vi "Scan_Hopping_percentDecrease_VUW.vi"() -> ()   [LabVIEW 2023]
uses:
  Sub_Vi/TypeDefs/Settings.ctl
  Sub_Vi/TypeDefs/ChangeOnFly.ctl
  Sub_Vi/TypeDefs/Display.ctl
  Settings.vi
panel:
  out "Precent Change for feedback (percent) 2":dbl=2.0
  in  "StopCond_GreaterThan? 2":bool
  in  "Display Cluster":T1
  in  "ChangeonFly":T2
  in  "SettingsCluster":T3={"Sample Rate (us)"=1, "Samples Per Data Point (int, power of 2)"=1000, "DistanceToBulk (um)"=-1.0, "HoldTimeScaler"=40000, "SaveData"=TRUE, "DistanceToBulk (um) 2"=-1.0, "DistanceToBulk (um) 3"=-1.0}
  in  "Feedback Type":T4(ring)=enum."Current 1"
  in  "StopCond_GreaterThan?":bool=TRUE
  in  "Approach Rate (um/s)":dbl=0.15
  in  "Retract Rate (um/s)":dbl=1.0
  in  "Hopping Distance (um)":dbl=1.0
  in  "Z End height (um)":dbl
  in  "Distance To Retract (um)":dbl=5.0
  in  "Upper dZ limit":i32=8
  in  "Precent Change for feedback (percent)":dbl=2.0
  in  "P":fxp<+/-,32,1>=0.029999999795109034 format="%.32g"
  in  "X Center (um)":dbl=100.0 min=0.0 max=300.0
  in  "Y Center (um)":dbl=100.0 min=0.0 max=300.0
  in  "Y Width (um)":dbl=10.0
  in  "X Width (um)":dbl=10.0
  in  "Scan Rate (um/s)":dbl=5.0
  in  "Voltage to Electrode (V)":dbl=-0.4
  in  "Z Start height (um)":dbl=150.0
  in  "Start scan Button":bool
  in  "Stop":bool
  in  "Pause":bool
  in  "Start Scanning Button":bool
  out "Y end":dbl
  out "X end":dbl
  out "X start":dbl
  out "Y start":dbl
  in  "Tab Control 4":enum32{"AC Approach 2"}(tab)
  out "t vs C1":dbl[](graph)
  out "Z vs C1":cluster{"Y":dbl[], "Y":dbl[]}[](graph)
  # "Approach  Settings"
  # "Feedback  Settings"
  # "Scan  Settings"
  # "Define Scan area \nAbout centre"
  # "Settings"
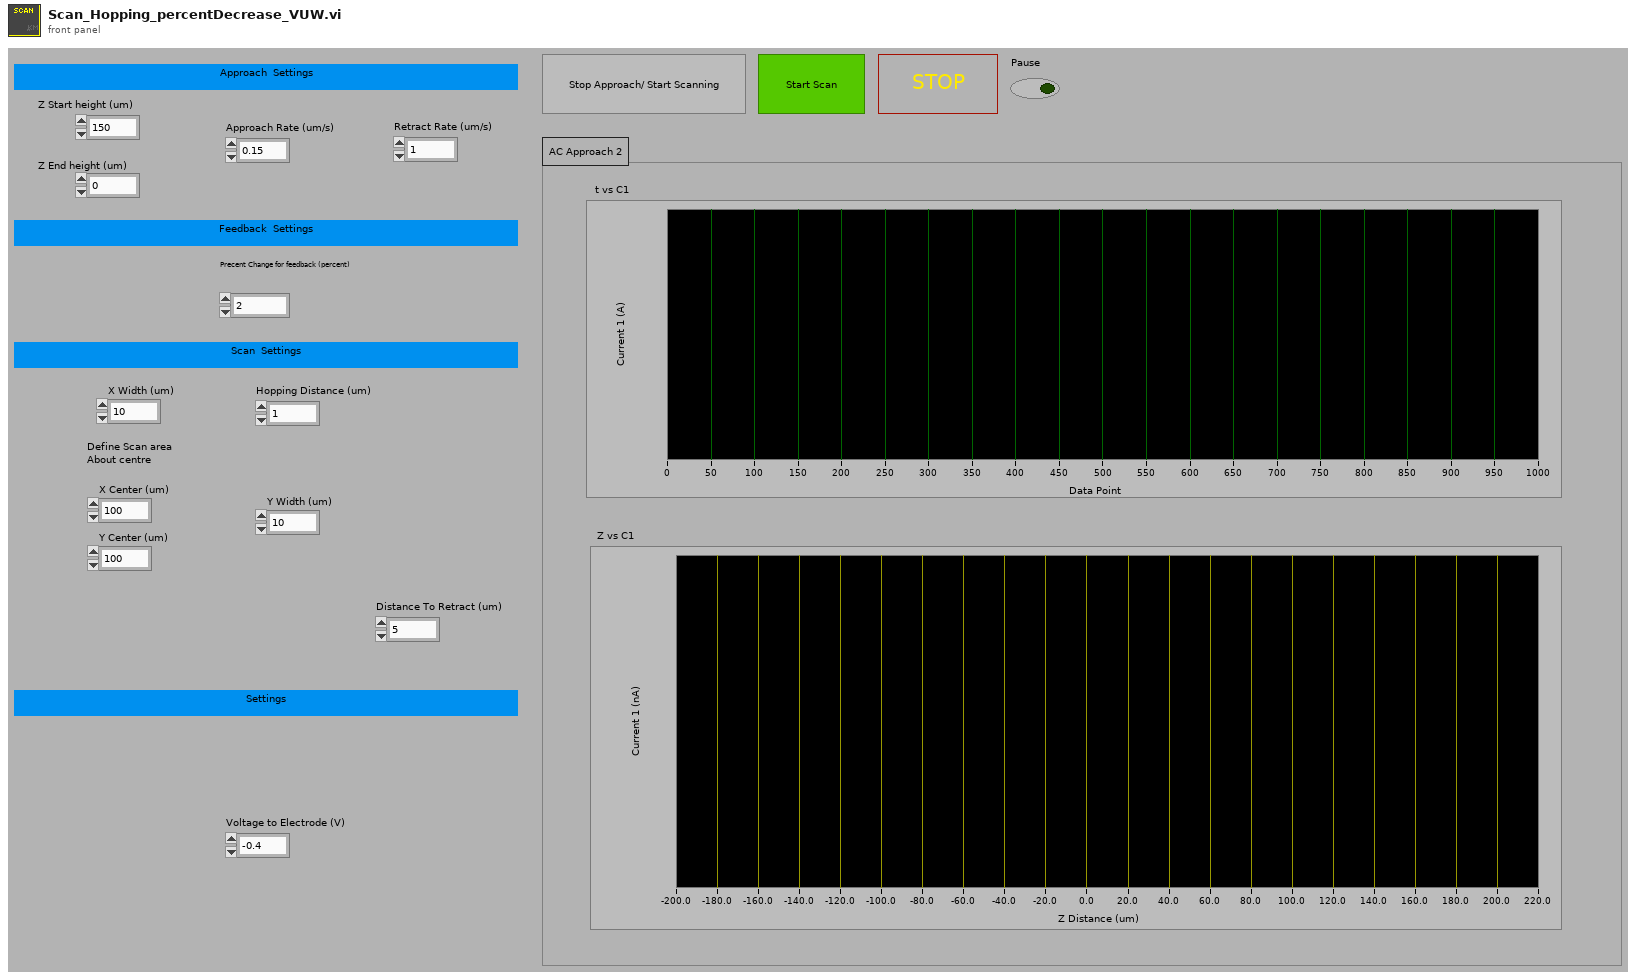
[diagram p1: front panel]
types:
  T1 = typedef "Display.ctl" = cluster{"X":refnum<vi>, "Y":refnum<vi>, "Z":refnum<vi>, "Amp":refnum<vi>, "Phase":refnum<vi>, "t vs Z":refnum<vi>, "t vs C1":refnum<vi>, "t vs C2":refnum<vi>, "t vs C3":refnum<vi>, "t vs Amp":refnum<vi>, "t vs Phase":refnum<vi>, "t vs X":refnum<vi>, "t vs Y":refnum<vi>, "Z vs C1":refnum<vi>, "Z vs C2":refnum<vi>, "Z vs C3":refnum<vi>, "V vs C1":refnum<vi>, "V vs C2":refnum<vi>, "V vs C3":refnum<vi>, "X/Y/Z F":refnum<vi>, "X/Y/Z R":refnum<vi>, "X/Y/C1 F":refnum<vi>, "X/Y/C1 R":refnum<vi>, "X/Y/C2 F":refnum<vi>, "X/Y/C2 R":refnum<vi>, "X/Y/C3 F":refnum<vi>, "X/Y/C3 R":refnum<vi>, "NumberOfLines":u16, "um Per Pixel":dbl, "um Per Line":dbl, "X Center":dbl, "Hop X/Y/Z":refnum<vi>, "Hop X/Y/C1":refnum<vi>, "Hop X/Y/C2":refnum<vi>, "Hop X/Y/C3":refnum<vi>, "X Width":dbl, "Y Width":dbl, "Hopping Distance":dbl, "V2 vs C1":refnum<vi>, "V vs Phase":refnum<vi>, "Y Center":dbl, "Number of Pixels":dbl, "V2 vs C2":refnum<vi>, "V2 vs C3":refnum<vi>, "V vs y":refnum<vi>, "V2 vs y":refnum<vi>, "Z vs Amp":refnum<vi>, "Z vs Phase":refnum<vi>}
  T2 = typedef "ChangeOnFly.ctl" = cluster{"Stop (boolean)":refnum<vi>, "Pause (boolean)":refnum<vi>, "EndCurrentLine (boolean)":refnum<vi>, "max movement per update step (Interger, nm)":refnum<vi>, "P (float, arb)":refnum<vi>, "Feedback set point (double, Amps)":refnum<vi>, "Voltage (double, V)":refnum<vi>, "Feedback set point 2 (double, Amps)":refnum<vi>, "Stop on Greater Than 2? (boolean)":refnum<vi>, "Stop on Greater Than? (boolean)":refnum<vi>, "Voltage 2 (double, V)":refnum<vi>, "Feedback Type (enum)":refnum<vi>, "Feedback Type 2 (enum)":refnum<vi>}
  T3 = typedef "Settings.ctl" = cluster{"Sample Rate (us)":u32, "Samples Per Data Point (int, power of 2)":i16, "DistanceToBulk (um)":dbl, "HoldTimeScaler":u64, "SaveData":bool, "DistanceToBulk (um) 2":dbl, "DistanceToBulk (um) 3":dbl}
  T4 = enum16{"AC Magnitude", "Current 1", "Current 2", "Phase"}
  T5 = cluster{"Scan Rate (um/s)":dbl, "X Start":dbl, "X End":dbl, "Y Start":dbl, "Y End":dbl, " Z Start":dbl, "HoppingDistance":dbl, "V":dbl, "Z End":dbl, "Approach Rate Hopping (um/s)":dbl, "Retrack Rate (um/s)":dbl, "V 2":dbl, "Approach Rate (um/s)":dbl, "Hold Time START / s":dbl, "Hold Time Delta / s":dbl, "Voltage to Electrode During Retract":dbl, "Pause on First Approach?":bool}
  T6 = typedef "Current Amplifier Settings.ctl" = dbl
  T7 = typedef "WayPointCluster.ctl" = cluster{"X (um)":dbl[], "Y (um)":dbl[], "Z (um)":dbl[], "V (V)":dbl[], "X Velocity (um s-1)":dbl[], "Y Velocity (um s-1)":dbl[], "Z Velocity (um s-1)":dbl[], "V Velocity (V s-1)":dbl[], "FeedBack Type (enum)":u16[], "Move X (boolean)":bool[], "Move Y (boolean)":bool[], "Move Z (boolean)":bool[], "Move V (boolean)":bool[], "Jump V (boolean)":bool[], "Hold (boolean)":bool[], "Hold Time":u32[], "V2 (V)":dbl[], "Move V2":bool[], "V2 Velocity (V s-1)":dbl[], "Jump V2 (boolean)":bool[], "Update z Position delta (ms)":i16[], "Hold Feedback1":bool[], "Move Z PicoMotor":bool[], " Z PicoMotor Direction":bool[], "DIO0":bool[]}
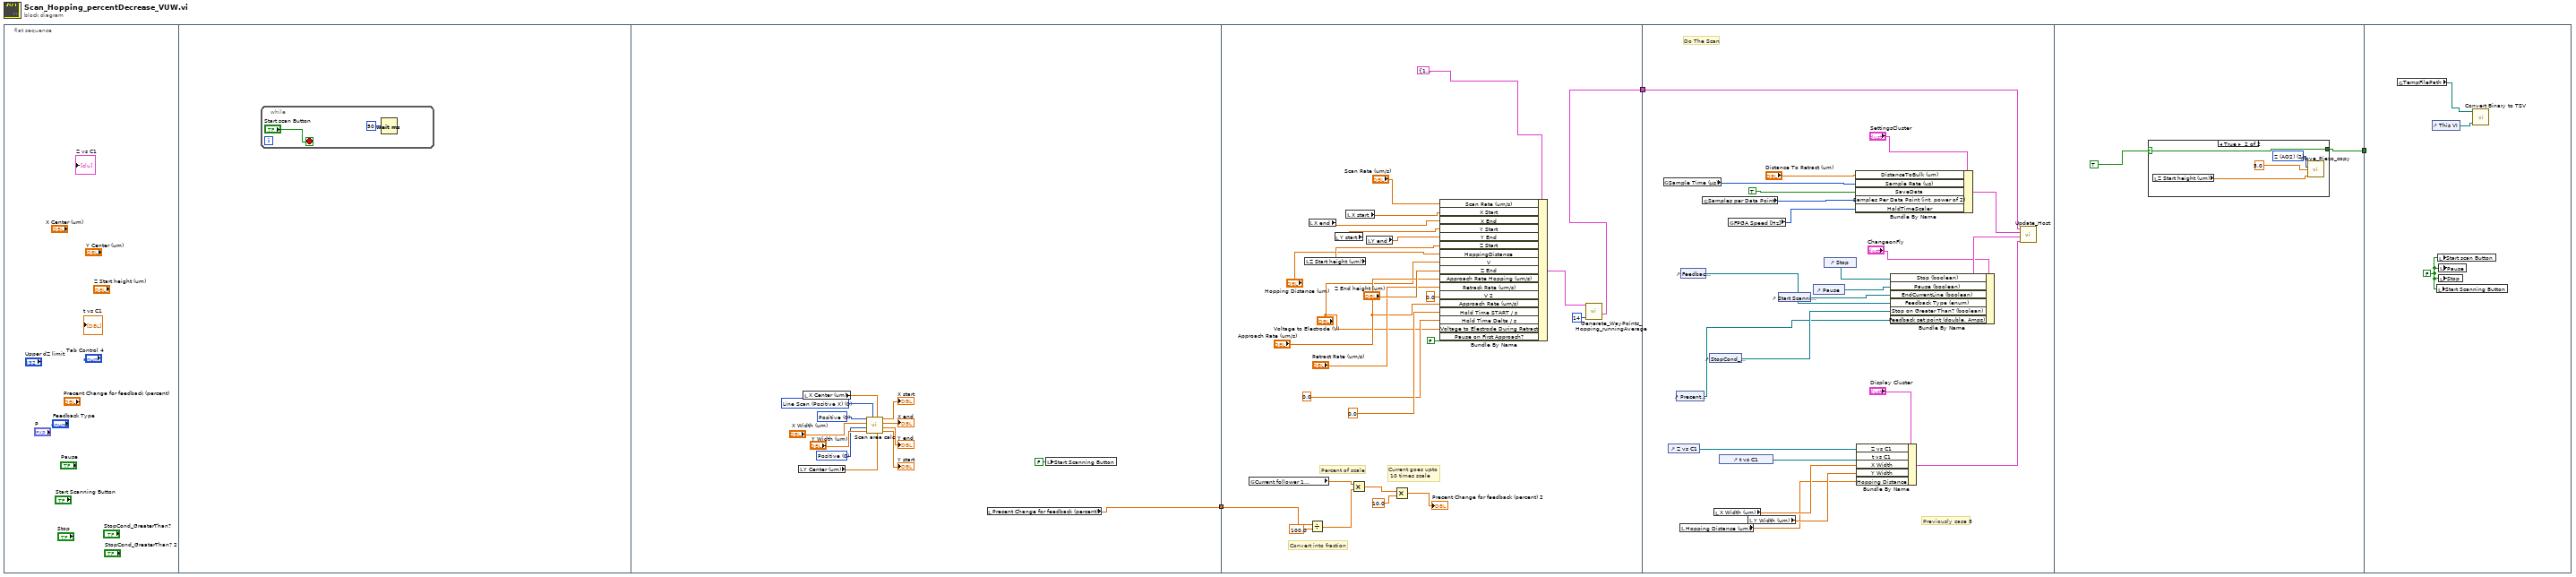
[diagram p0: block diagram]
diagram:
  n1 = flat-sequence {
    tunnel: [w6] -> w1
    tunnel: [w27] -> w3
    tunnel: w1 -> [w25]
    tunnel: w3 -> [w67]
    tunnel: [w68] -> w2
    tunnel: w2 -> [_]
    frame #0 {
    }
    frame #1 {
      n2 = while {
        stop <- "Start scan Button" stop-if-true
        n3 = Wait (ms)(milliseconds to wait=u32 50) -> ()  [unwired: 1 out]
      }
    }
    frame #2 {
      w10 = u16 0 items=["Positive", "Negative"] ("Major Axis Direction")
      w9 = u16 0 items=["Positive", "Negative"] ("Minor Axis Direction")
      w8 = u16 0 items=["Line Scan (Positive X)", "Line Scan (Negative X)", "Line Scan (Positive Y)", "Line Scan (Negative Y)"] ("Scan Type")
      n4 = local read "Y Center (um)"() -> (w18:dbl)
      n5 = local read "X Center (um)"() -> (w17:dbl)
      n6 = call "Scan area calc.vi"("Y Width"="Y Width (um)", "Major Axis Direction"=w10, "X Width"="X Width (um)", "Minor Axis Direction"=w9, "Scan Type"=w8, "Y Center"=w18, "X Center"=w17) -> ("Y start"=→"Y start":dbl, "Y end"=→"Y end":dbl, "X end"=→"X end":dbl, "X start"=→"X start":dbl)
      n7 = local read "Precent Change for feedback (percent)"() -> (w6:dbl)
      n8 = local write "Start Scanning Button"(FALSE ("Start Scanning Button")) -> ()
    }
    frame #3 {
      # "Current goes upto\n 10 times scale"
      # "Percent of scale"
      # "Convert into fraction"
      n9 = global read "Settings.vi" "Current follower 1\n (AI-3)"() -> (w22:T6)
      n10 = local read "Z Start height (um)"() -> (w38:dbl)
      n11 = local read "X end"() -> (w41:dbl)
      n12 = Divide(x=w25, y=100.0) -> (x/y=w23:dbl)
      n13 = local read "Y start"() -> (w40:dbl)
      n14 = local read "X start"() -> (w42:dbl)
      n15 = Multiply(x=w22, y=w23) -> (x*y=w21:T6)
      n16 = local read "Y end"() -> (w39:dbl)
      n17 = Multiply(x=w21, y=10.0) -> (x*y=→"Precent Change for feedback (percent) 2":T6)
      n18 = Bundle By Name(cluster=T5 {"Scan Rate (um/s)"=15.0, "X Start"=15.0, "X End"=15.0, "Y Start"=15.0, "Y End"=15.0, " Z Start"=15.0, "HoppingDistance"=1.0, "V"=15.0, "Z End"=15.0, "Approach Rate Hopping (um/s)"=15.0, "Retrack Rate (um/s)"=15.0, "V 2"=15.0, "Approach Rate (um/s)"=15.0, "Hold Time START / s"=15.0, "Hold Time Delta / s"=15.0, "Voltage to Electrode During Retract"=0.0, "Pause on First Approach?"=FALSE} ("Input Cluster"), "Scan Rate (um/s)"="Scan Rate (um/s)", "X Start"=w42, "X End"=w41, "Y Start"=w40, "Y End"=w39, "Z Start"=w38, "HoppingDistance"="Hopping Distance (um)", "V"="Voltage to Electrode (V)", "Z End"="Z End height (um)", "Approach Rate Hopping (um/s)"="Approach Rate (um/s)", "Retrack Rate (um/s)"="Retract Rate (um/s)", "V 2"=0.0, "Approach Rate (um/s)"="Approach Rate (um/s)", "Hold Time START / s"=0.0 ("IT Time /s"), "Hold Time Delta / s"=0.0 ("IT Time Delta /s"), "Voltage to Electrode During Retract"="Voltage to Electrode (V)", "Pause on First Approach?"=FALSE) -> (w28:T5)
      n19 = call "Generate_WayPoints_Hopping_runningAverage.vi"("element"=u16 14, "Input Cluster"=w28) -> ("output cluster"=w27:T7)  [unwired: 9 in]
    }
    frame #4 {
      # "Previously case 8"
      # "Do The Scan"
      n20 = global read "Settings.vi" "Sample Time (µs)"() -> (w50:u32)
      n21 = control-ref of="Z vs C1"() -> (w59:refnum<vi>)
      n22 = control-ref of="Precent Change for feedback (percent) 2"() -> (w45:refnum<vi>)
      n23 = local read "Hopping Distance (um)"() -> (w56:dbl)
      n24 = control-ref of="Feedback Type"() -> (w48:refnum<vi>)
      n25 = global read "Settings.vi" "Samples per Data Point"() -> (w52:u16)
      n26 = control-ref of="StopCond_GreaterThan?"() -> (w47:refnum<vi>)
      n27 = local read "X Width (um)"() -> (w58:dbl)
      n28 = control-ref of="t vs C1"() -> (w60:refnum<vi>)
      n29 = global read "Settings.vi" "FPGA Speed [Hz]"() -> (w46:i64)
      n30 = local read "Y Width (um)"() -> (w57:dbl)
      n31 = control-ref of="Start Scanning Button"() -> (w63:refnum<vi>)
      n32 = control-ref of="Pause"() -> (w62:refnum<vi>)
      n33 = control-ref of="Stop"() -> (w61:refnum<vi>)
      n34 = Bundle By Name(cluster="SettingsCluster", "DistanceToBulk (um)"="Distance To Retract (um)", "Sample Rate (us)"=w50, "SaveData"=TRUE ("Save Data"), "Samples Per Data Point (int, power of 2)"=w52, "HoldTimeScaler"=w46) -> (w65:T3)
      n35 = Bundle By Name(cluster="Display Cluster", "Z vs C1"=w59, "t vs C1"=w60, "X Width"=w58, "Y Width"=w57, "Hopping Distance"=w56) -> (w66:T1)
      n36 = Bundle By Name(cluster="ChangeonFly", "Stop (boolean)"=w61, "Pause (boolean)"=w62, "EndCurrentLine (boolean)"=w63, "Feedback Type (enum)"=w48, "Stop on Greater Than? (boolean)"=w47, "Feedback set point (double, Amps)"=w45) -> (w64:T2)
      n37 = call "Update_Host.vi"("Display Cluster"=w66, "ChangeonFly"=w64, "SettingsCluster"=w65, "WayPointCluster"=w67) -> ()  [unwired: 6 in]
    }
    frame #5 {
      n38 = case shown="True" TRUE ("Retract after approach over (T/F)") {
        selector: TRUE ("Retract after approach over (T/F)") -> [w70 w71]
        tunnel: [w70 w71] -> w68
        frame False {
        }
        frame True {
          w74 = u16 2 items=["X (AO0)", "Y (AO1)", "Z (AO2)", "V (AO3)"] ("Channel")
          n39 = local read "Z Start height (um)"() -> (w72:dbl)
          n40 = call "Move_Piezo_copy.vi"("Piezo"=w74, "Movement Speed (µm/s)"=5.0 ("Scan Rate (um/s)"), "Position (µm) (or V)"=w72) -> ()  [unwired: 13 in]
        }
      }
    }
    frame #6 {
      w77 = FALSE ("Stop")
      n41 = global read "Settings.vi" "TempFilePath"() -> (w75:path)
      n42 = control-ref of="This VI"() -> (w76:refnum<vi>)
      n43 = local write "Start Scanning Button"(w77) -> ()
      n44 = local write "Start scan Button"(w77) -> ()
      n45 = local write "Pause"(w77) -> ()
      n46 = local write "Stop"(w77) -> ()
      n47 = call "Convert Binary to TSV.vi"("This VI"=w76, "TDMS DataFile Name"=w75) -> ()  [unwired: 10 in]
    }
  }
